vi "test Acyclic Loopback Multiple Pretrigger Writes.vi"(8 "error in":errorcluster, 11 "TestCase in":refnum<class "Single Board Loopback.lvclass">) -> (0 "error out":errorcluster, 3 "TestCase out":refnum<class "Single Board Loopback.lvclass">)   [LabVIEW 2020, in "Single Board Loopback.lvclass"]
uses:
  Single Board Loopback.lvclass
  <vilib>/addons/_JKI Toolkits/VI Tester/TestCase.llb/TestCase.lvclass
  <vilib>/NI VeriStand/Execution/Workspace/NI_VS Workspace ExecutionAPI.lvlib
  niveristand-custom-device-testing-tools/VeriStandTestUtilities/VeriStandTestUtilities.lvlib
  <vilib>/NI VeriStand/Execution/Workspace/NI VeriStand - Set Multiple Channel Values.vi
  <vilib>/numeric/Random Number (Range) U64.vi
  C:/Users/nitest/Desktop/Git 2020/niveristand-custom-device-testing-tools/VeriStandTestCase/VeriStandTestCase.lvclass
  C:/Program Files (x86)/National Instruments/LabVIEW 2020/vi.lib/addons/_JKI Toolkits/VI Tester/TestCase.llb/TestCase.lvclass
  C:/Users/nitest/Desktop/Git 2020/niveristand-ballard-arinc429-custom-device/Source/Custom Device Support/Tests/System/Single Board Loopback/Single Board Loopback.lvclass
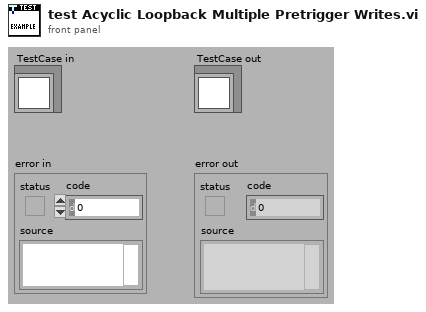
[diagram p1: front panel]
types:
  T1 = typedef "NI_VS Workspace ExecutionAPI.lvlib/WorkspaceAPI.ctl" = refnum<k24>
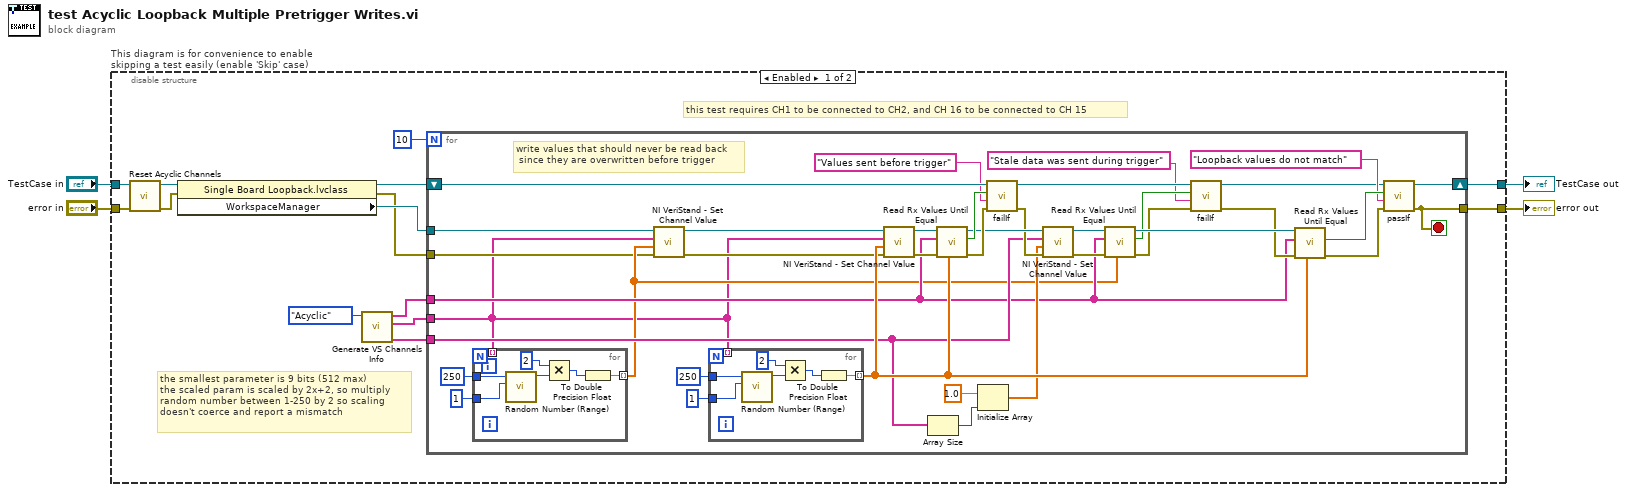
[diagram p0: block diagram]
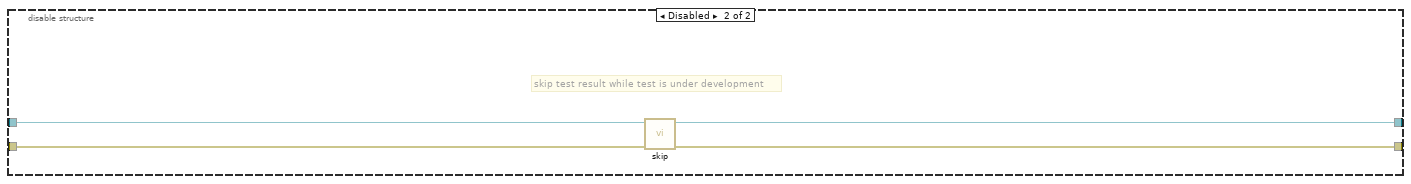
[diagram p2: hidden frame]
diagram:
  n1 = disable-structure "This diagram is for convenience to enable skipping a test easily (enable 'Skip' case)" shown="Enabled" {
    disable-tunnel: "TestCase in" -> [w5 w72]
    disable-tunnel: [w12 w70] -> w1
    disable-tunnel: [w11 w71] -> w3
    disable-tunnel: "error in" -> [w13 w69]
    frame Enabled {
      # "the smallest parameter is 9 bits (512 max)\nthe scaled param is scaled by 2x+2, so multiply \nrandom number between 1-250 by 2 so scaling\ndoesn't coerce and report a mismatch"
      # "this test requires CH1 to be connected to CH2, and CH 16 to be connected to CH 15"
      n2 = call "Reset Acyclic Channels.vi"("error in (no error)"=w13, "reference in"=w5) -> ("error out"=w7:errorcluster, "reference out"=w6:refnum<class "Single Board Loopback.lvclass">)  [unwired: 8 in]
      n3 = property class="Single Board Loopback.lvclass"(reference=w6, error in=w7) -> (reference out=w15:refnum<class "Single Board Loopback.lvclass">, error out=w16:errorcluster, "WorkspaceManager"=w17:T1)
      n4 = call "Generate VS Channels Info.vi"("Transfer Type"=enum16{"Acyclic", "Scheduled"}."Acyclic") -> ("Tx Trigger Channels Array"=w9:string[], "Tx Channels Array"=w10:string[], "Rx Channels Array"=w18:string[])  [unwired: 6 in, 2 out]
      n5 = for {
        N: 10 -> [_]
        tunnel: w18 -> [w26]
        tunnel: w17 -> [w23]
        tunnel: w16 -> [w20]
        tunnel: w10 -> [w19]
        shift-right: [w44] -> w12
        shift-left: w15 -> [w51]
        tunnel: [w43] -> w11
        tunnel: w9 -> [w38]
        stop <- w43 stop-if-true
        # "write values that should never be read back\n since they are overwritten before trigger"
        n6 = for {
          tunnel: [w61] -> w25 mode=indexing
          tunnel: u64 250 ("upper bound (100)") -> [w60]
          tunnel: u64 1 ("upper bound (100)") -> [w59]
          tunnel: w19 -> [_] mode=indexing
          n7 = call-poly <vilib>:"Random Number (Range).vi"("lower bound (0)"=w59, "upper bound (100)"=w60) -> ("number"=w62:u64)  [unwired: 9 in]
          n8 = Multiply(x=u64 2, y=w62) -> (x*y=w58:u64)
          n9 = To Double Precision Float(number=w58) -> (double precision float=w61:dbl)
        }
        n10 = call-poly <vilib>:"NI VeriStand - Set Channel Value.vi"("error in (no error)"=w20, "Values"=w25, "Channels"=w19, "WorkspaceManager in"=w23) -> ("error out"=w21:errorcluster, "WorkspaceManager out"=w22:T1)  [unwired: 6 in]
        n11 = for {
          tunnel: [w67] -> w47 mode=indexing
          tunnel: u64 250 ("upper bound (100)") -> [w66]
          tunnel: u64 1 ("upper bound (100)") -> [w65]
          tunnel: w19 -> [_] mode=indexing
          n12 = call-poly <vilib>:"Random Number (Range).vi"("lower bound (0)"=w65, "upper bound (100)"=w66) -> ("number"=w68:u64)  [unwired: 9 in]
          n13 = Multiply(x=u64 2, y=w68) -> (x*y=w64:u64)
          n14 = To Double Precision Float(number=w64) -> (double precision float=w67:dbl)
        }
        n15 = call-poly <vilib>:"NI VeriStand - Set Channel Value.vi"("error in (no error)"=w21, "Values"=w47, "Channels"=w19, "WorkspaceManager in"=w22) -> ("error out"=w52:errorcluster, "WorkspaceManager out"=w54:T1)  [unwired: 6 in]
        n16 = Array Size(array=w38) -> (size(s)=w37:i32)
        n17 = call "Read Rx Values Until Equal.vi"("expected values"=w47, "error in"=w52, "Rx aliases"=w26, "workspace manager in"=w54) -> ("error out"=w53:errorcluster, "values equal expected"=w50:bool, "workspace manager out"=w49:T1)  [unwired: 5 in]
        n18 = Initialize Array(1.0, w37) -> (w39:dbl[])
        n19 = call-dynamic "failIf.vi"("error in (no error)"=w53, "message (\"\")"="Values sent before trigger" ("message (\"\")"), "fail"=w50, "TestCase in"=w51) -> ("error out"=w48:errorcluster, "TestCase out"=w31:refnum<class "Single Board Loopback.lvclass">)  [unwired: 6 in]
        n20 = call-poly <vilib>:"NI VeriStand - Set Channel Value.vi"("error in (no error)"=w48, "Values"=w39, "Channels"=w38, "WorkspaceManager in"=w49) -> ("error out"=w34:errorcluster, "WorkspaceManager out"=w33:T1)  [unwired: 6 in]
        n21 = call "Read Rx Values Until Equal.vi"("expected values"=w25, "error in"=w34, "Rx aliases"=w26, "workspace manager in"=w33) -> ("error out"=w29:errorcluster, "values equal expected"=w27:bool, "workspace manager out"=w32:T1)  [unwired: 5 in]
        n22 = call-dynamic "failIf.vi"("error in (no error)"=w29, "message (\"\")"="Stale data was sent during trigger" ("message (\"\")"), "fail"=w27, "TestCase in"=w31) -> ("error out"=w28:errorcluster, "TestCase out"=w30:refnum<class "Single Board Loopback.lvclass">)  [unwired: 6 in]
        n23 = call "Read Rx Values Until Equal.vi"("expected values"=w47, "error in"=w28, "Rx aliases"=w26, "workspace manager in"=w32) -> ("error out"=w45:errorcluster, "values equal expected"=w46:bool)  [unwired: 5 in, 1 out]
        n24 = call-dynamic "passIf.vi"("error in (no error)"=w45, "message (\"\")"="Loopback values do not match" ("message (\"\")"), "pass"=w46, "TestCase in"=w30) -> ("error out"=w43:errorcluster, "TestCase out"=w44:refnum<class "Single Board Loopback.lvclass">)  [unwired: 6 in]
      }
    }
    frame Disabled {
      # "skip test result while test is under development"
      n25 = call <vilib>:"skip.vi"("error in (no error)"=w69, "TestCase in"=w72) -> ("error out"=w71:errorcluster, "TestCase out"=w70:refnum<class "Single Board Loopback.lvclass">)  [unwired: 8 in]
    }
  }
  "error out" <- w3
  "TestCase out" <- w1
